vi "Status mit GD Info aktualisieren.vi"(7 "show Status even if no Error":bool, 8 "error in (no error)":errorcluster caption="Fehler (Eingang, kein Fehler)", 10 "Sprachliste":string[][](array[string]), 11 "GD Info-Cluster in":T1) -> (0 "error out":errorcluster caption="Fehler (Ausgang)", 3 "Status out":string)   [LabVIEW 2020, in "Linearisierung v2.lvlib" / "SpanEinstellungen.lvlib"]
uses:
  SpanEinstellungen.lvlib
  GD Info Cluster.ctl
  LIN ErrorCluster.ctl
  Gasteiler/Aktion FGV Daten Abholung uebergebenctl.ctl
  Gasteiler/Gasteiler.lvlib
  Allgemein/allgemeine Sub-VIs.lvlib
  Linearisierung v2.lvlib
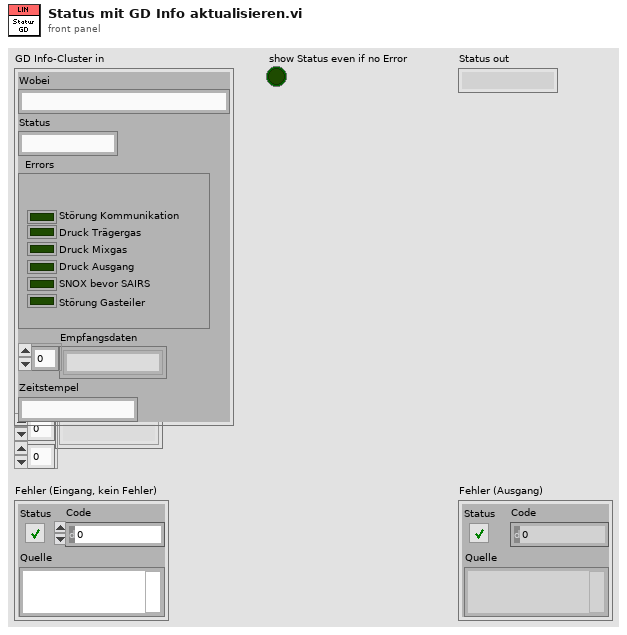
[diagram p1: front panel]
types:
  T1 = typedef "Linearisierung v2.lvlib/SpanEinstellungen.lvlib/GD Info Cluster.ctl" = cluster{"Wobei":string, "Status":string, "Errors":T2, "Empfangsdaten":string[], "Zeitstempel":string}
  T2 = typedef "Linearisierung v2.lvlib/LIN ErrorCluster.ctl" = cluster{"Störung Kommunikation":bool, "Pressure carrier gas":bool, "Pressure diluted gas":bool, "Outlet Pressure":bool, "SNOX before SAIR":bool, "Störung Gasteiler":bool}
  T3 = typedef "Linearisierung v2.lvlib/Gasteiler.lvlib/Aktion FGV Daten Abholung uebergebenctl.ctl" = enum16{"lesen", "schreiben", "Anzeigebit löschen", "Status hinzufügen"}
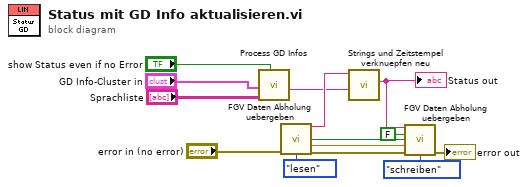
[diagram p0: block diagram]
diagram:
  n1 = call "Process GD Infos.vi"("show Status even if no Error"="show Status even if no Error", "Sprachliste"="Sprachliste", "GD Info-Cluster in"="GD Info-Cluster in") -> ("GD Infos"=w4:string)  [unwired: 6 in, 2 out]
  n2 = call "FGV Daten Abholung uebergeben.vi"("error in (no error)"="error in (no error)", "Aktion"=Aktion_FGV_Daten_Abholung_uebergebenctl."lesen") -> ("Zustand"=w7:string, "Beendet"=w8:bool, "Restlaufzeit out"=w9:sgl, "error out"=w10:errorcluster)  [unwired: 9 in, 1 out]
  n3 = call "Strings und Zeitstempel verknuepfen neu.vi"("String 1 hinzufügen"=w4, "Eingangs String"=w7) -> ("Verknüpfter String"=w6:string)  [unwired: 9 in]
  "Status out" <- w6
  n4 = call "FGV Daten Abholung uebergeben.vi"("Zustand"=w6, "Anzeige aktualisieren"=FALSE, "Beendet"=w8, "Restlaufzeit"=w9, "error in (no error)"=w10, "Aktion"=Aktion_FGV_Daten_Abholung_uebergebenctl."schreiben") -> ("error out"=→"error out":errorcluster)  [unwired: 5 in, 4 out]
